vi "Hall of 6-Contact Sample Test.vi"(8 "error in (no error)":errorcluster) -> (0 "error out":errorcluster)   [LabVIEW 2016, in "Hall Effect Library.lvlib"]
uses:
  Hall Effect Library.lvlib
  Controls/Measurement.ctl
  Public/Controls/Data Items.ctl
  Public/Controls/Tests.ctl
  Global Variables/Test Settings.vi
  Global Variables/Hall Effect Data.vi
  Global Variables/Instrument Locations.vi
panel:
  out "Test Step":T1(ring)
  out "Measurement":T2
  out "Soak Until":timestamp
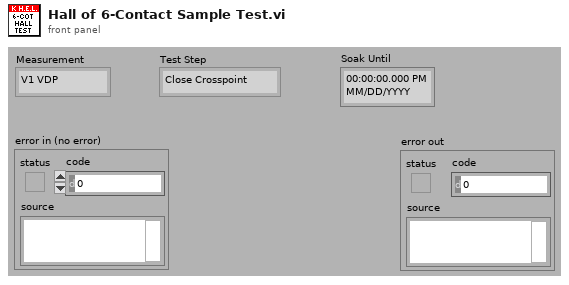
[diagram p1: front panel]
types:
  T1 = enum16{"Close Crosspoint", "Soak 1", "Zero Ammeter", "Zero Voltmeter", "I-SRC On", "Init Ammeter", "Soak 2", "Measure I", "Measure V", "I-SRC Off", "Open Crosspoint", "Done"}
  T2 = typedef "Hall Effect Library.lvlib/Measurement.ctl" = enum16{"V1 VDP", "V2 VDP", "V3 VDP", "V4 VDP", "V5 VDP", "V6 VDP", "V7 VDP", "V8 VDP", "V1 HE", "V2 HE", "V3 HE", "V4 HE", "V5 HE", "V6 HE", "V7 HE", "V8 HE", "V1 Res Bar", "V1 Hall Bar", "V1 Res 6-Cot", "V2 Res 6-Cot", "V3 Res 6-Cot", "V4 Res 6-Cot", "V1 Hall 6-Cot", "V2 Hall 6-Cot", "V3 Hall 6-Cot", "V4 Hall 6-Cot", "V5 Hall 6-Cot", "V6 Hall 6-Cot", "V7 Hall 6-Cot", "V8 Hall 6-Cot", "V1 Res 8-Cot", "V2 Res 8-Cot", "V3 Res 8-Cot", "V4 Res 8-Cot", "V1 Hall 8-Cot", "V2 Hall 8-Cot", "V3 Hall 8-Cot", "V4 Hall 8-Cot"}
  T3 = cluster{"RAvg":dbl, "RH1":dbl, "RH2":dbl, "uH":dbl}
  T4 = typedef "Hall Effect Library.lvlib/Resisitivity.ctl" = enum16{"Low", "High"}
  T5 = typedef "Hall Effect Library.lvlib/Tests.ctl" = enum16{"Van Der Pauw", "Hall Effect", "Bar Sample Resistivity", "Bar Sample Hall ", "6-Contact Sample Resistivity", "6-Contact Sample Hall", "8-Contact Sample Resistivity", "8-Contact Sample Hall", ""}
  T6 = typedef "Hall Effect Library.lvlib/Data Items.ctl" = enum16{"V1 Van Der Pauw", "V2 Van Der Pauw", "V3 Van Der Pauw", "V4 Van Der Pauw", "V5 Van Der Pauw", "V6 Van Der Pauw", "V7 Van Der Pauw", "V8 Van Der Pauw", "V1 Hall Effect", "V2 Hall Effect", "V3 Hall Effect", "V4 Hall Effect", "V5 Hall Effect", "V6  Hall Effect", "V7 Hall Effect", "V8 Hall Effect", "V1 Res Bar", "V1 Hall Bar", "V1 Res 6-Cot", "V2 Res 6-Cot", "V3 Res 6-Cot", "V4 Res 6-Cot", "V1 Hall 6-Cot", "V2 Hall 6-Cot", "V3 Hall 6-Cot", "V4 Hall 6-Cot", "V5 Hall 6-Cot", "V6 Hall 6-Cot", "V7 Hall 6-Cot", "V8 Hall 6-Cot", "V1 Res 8-Cot", "V2 Res 8-Cot", "V3 Res 8-Cot", "V4 Res 8-Cot", "V1 Hall 8-Cot", "V2 Hall 8-Cot", "V3 Hall 8-Cot", "V4 Hall 8-Cot", "Van Der Pauw Results", "Hall Effect Results", "Bar Sample Resistivity Results", "Bar Sample Hall Results", "6-Contact Resistivity Results", "6-Contact Hall Results", "8-Contact Resistivity Results", "8-Contact Hall Results"}
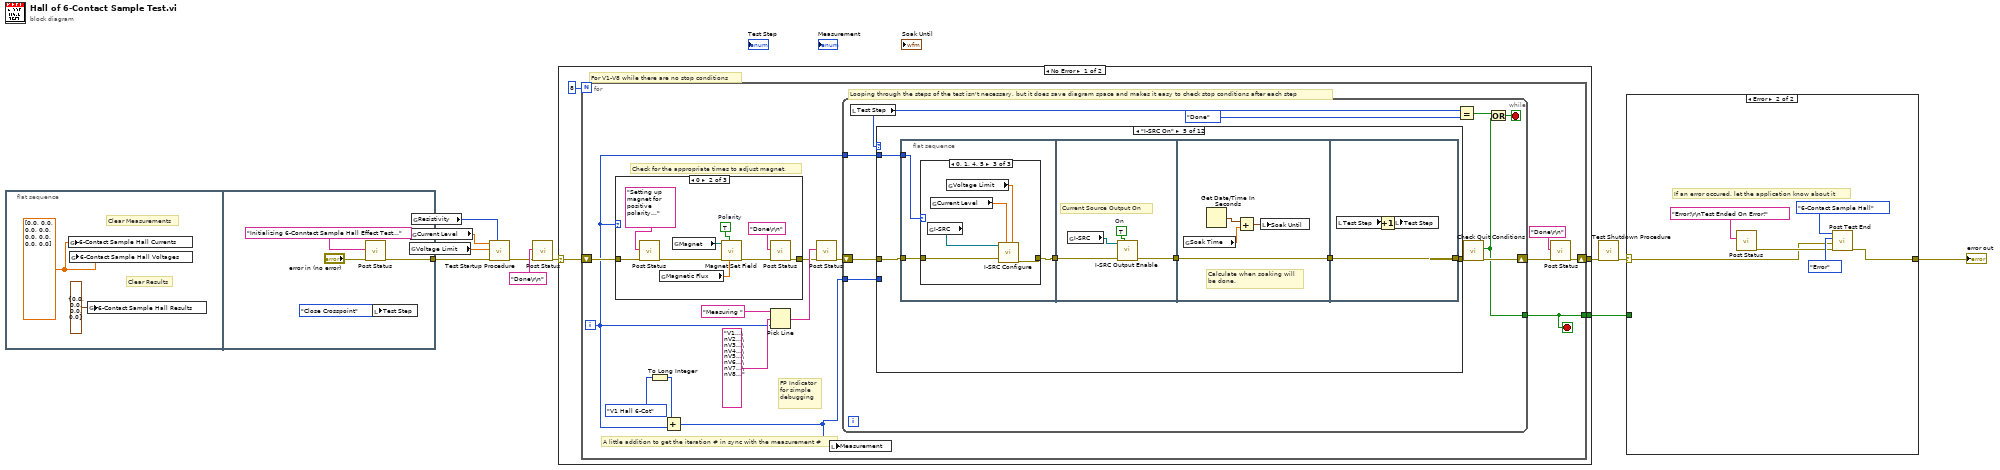
[diagram p0: block diagram]
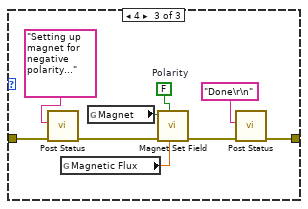
[diagram p3: hidden frame]
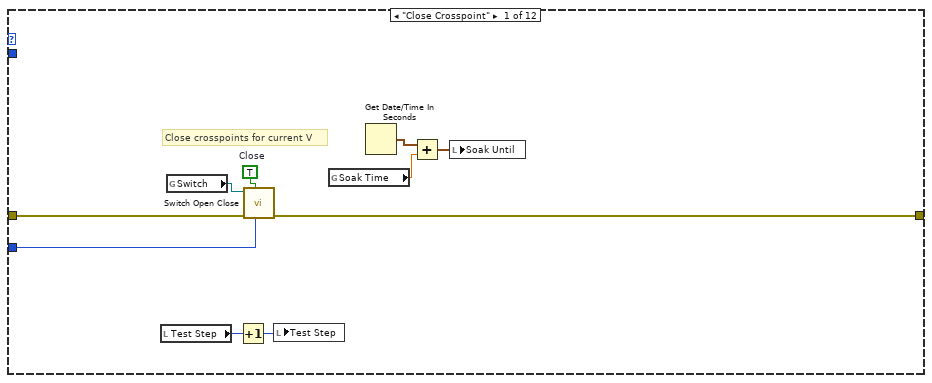
[diagram p4: hidden frame]
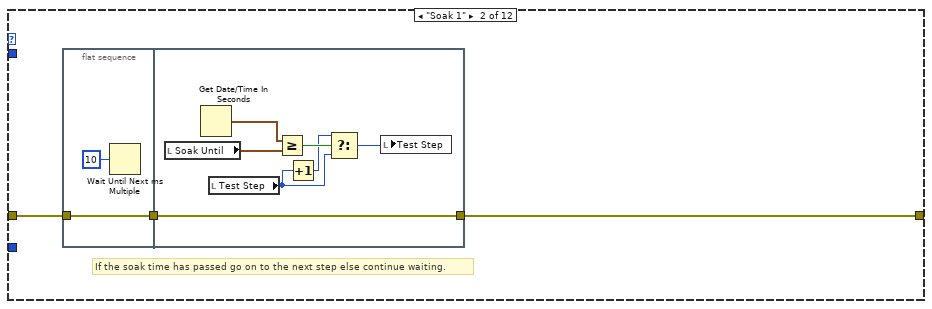
[diagram p5: hidden frame]
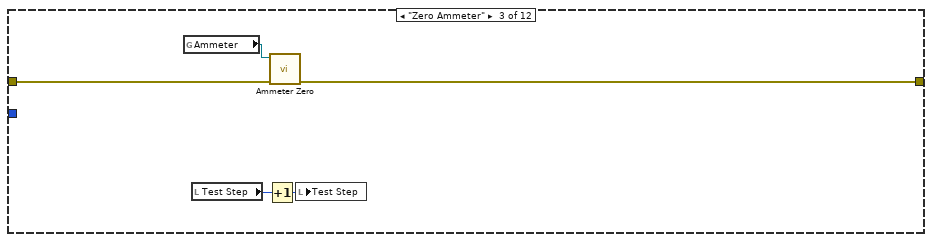
[diagram p6: hidden frame]
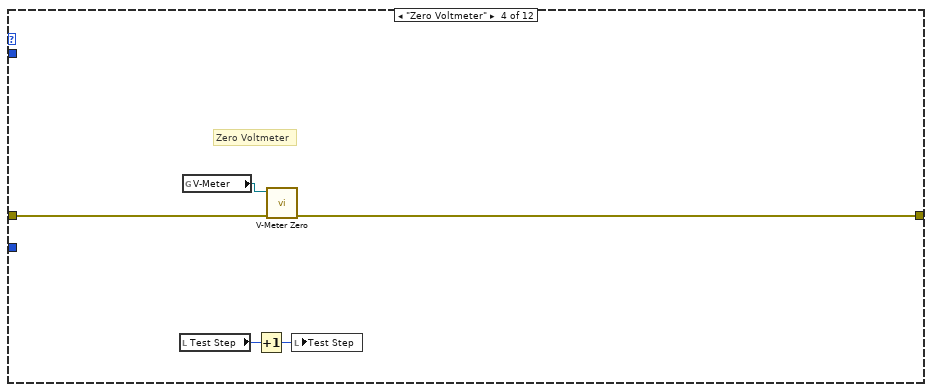
[diagram p7: hidden frame]
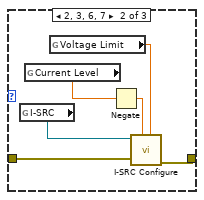
[diagram p9: hidden frame]
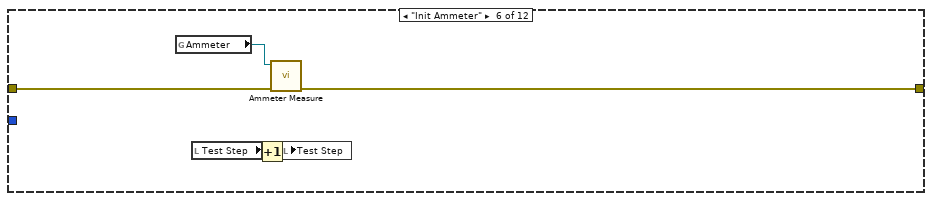
[diagram p10: hidden frame]
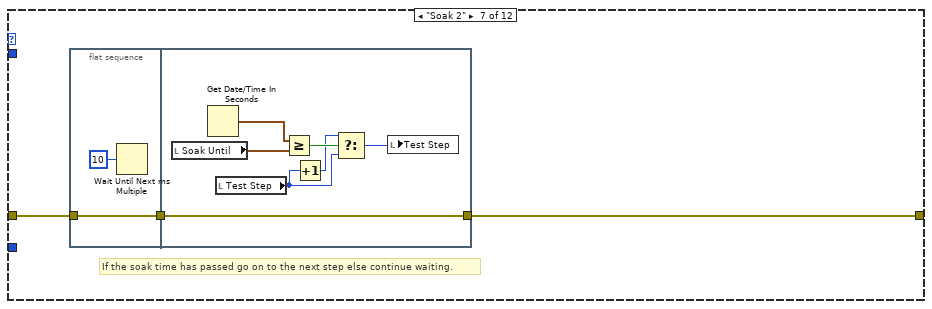
[diagram p11: hidden frame]
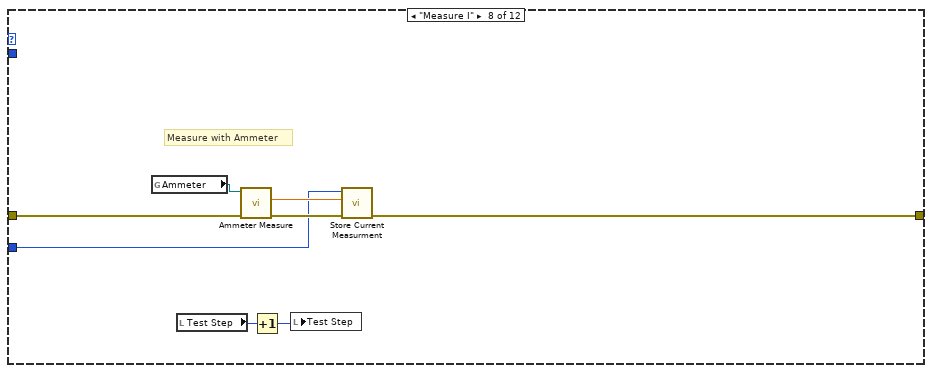
[diagram p12: hidden frame]
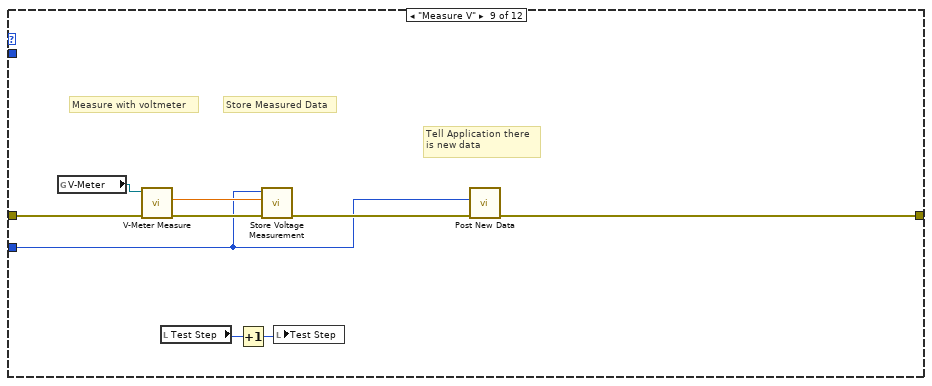
[diagram p13: hidden frame]
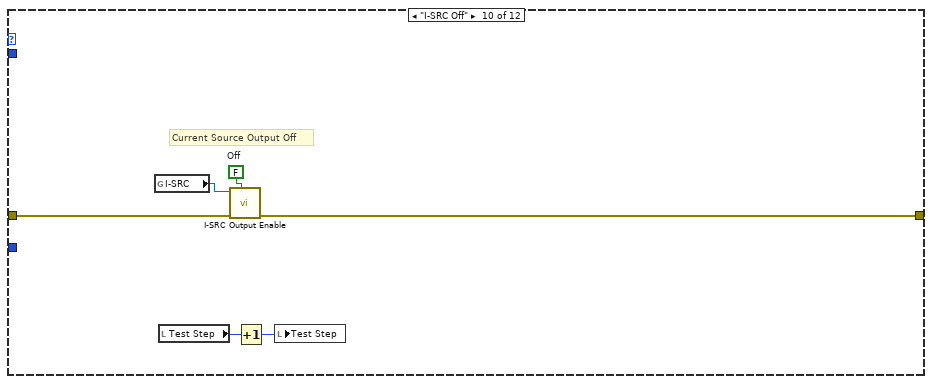
[diagram p14: hidden frame]
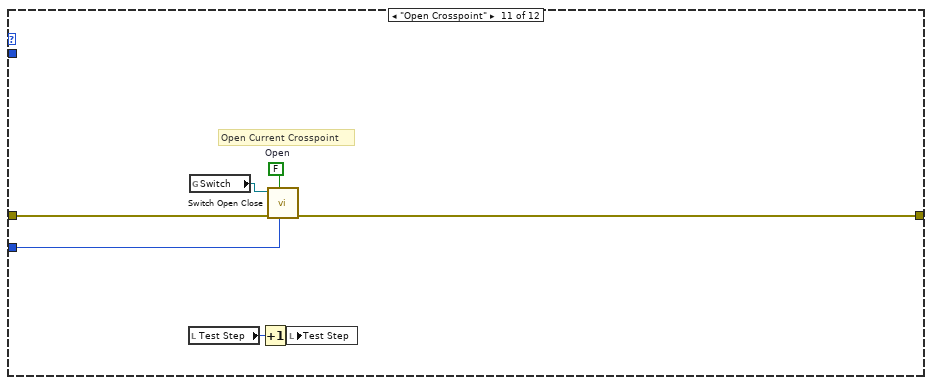
[diagram p15: hidden frame]
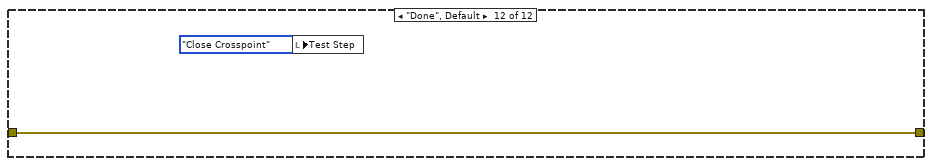
[diagram p16: hidden frame]
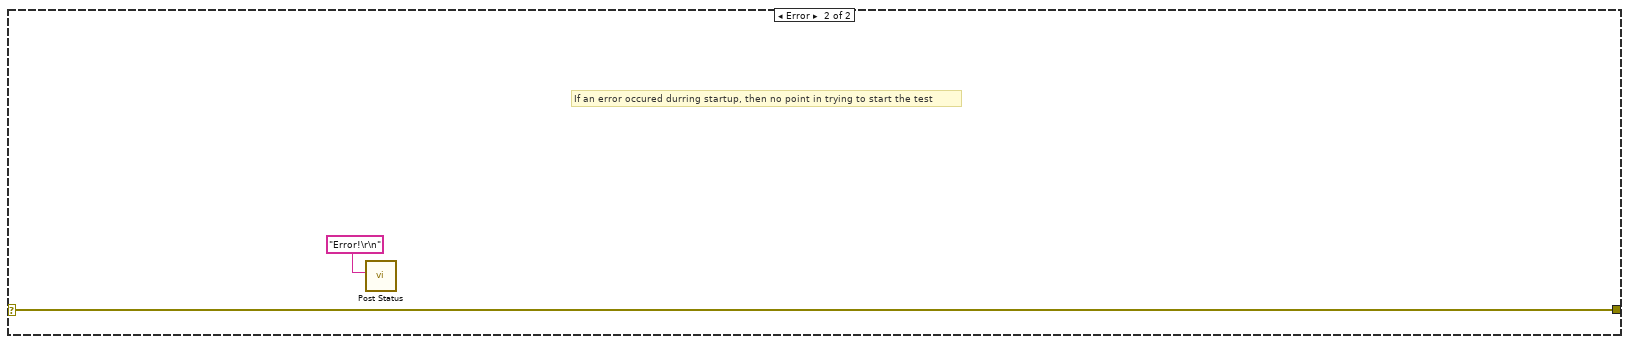
[diagram p17: hidden frame]
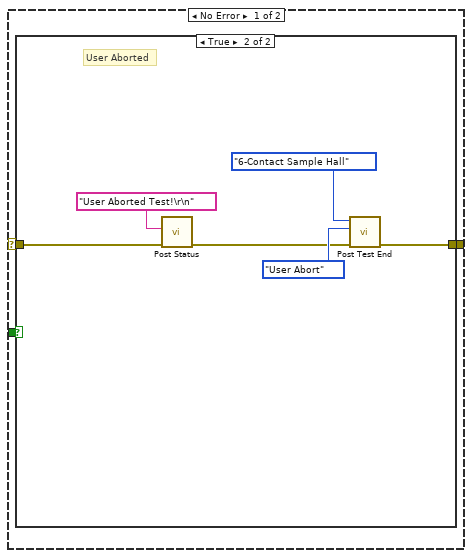
[diagram p18: hidden frame]
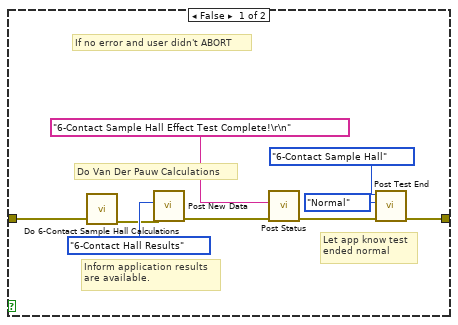
[diagram p19: hidden frame]
diagram:
  n1 = flat-sequence {
    tunnel: [w17] -> w5
    frame #0 {
      w12 = dbl[] [0.0, 0.0, 0.0, 0.0, 0.0, 0.0, 0.0, 0.0] ("6-Contact Sample Hall Voltages")
      # "Clear Results"
      # "Clear Measurements"
      n2 = global write "Hall Effect Data.vi" "6-Contact Sample Hall Currents"(w12) -> ()
      n3 = global write "Hall Effect Data.vi" "6-Contact Sample Hall Voltages"(w12) -> ()
      n4 = global write "Hall Effect Data.vi" "6-Contact Sample Hall Results"(T3 {"RAvg"=0.0, "RH1"=0.0, "RH2"=0.0, "uH"=0.0} ("6-Contact Sample Hall Results")) -> ()
    }
    frame #1 {
      n5 = call "Post Status.vi"("error in (no error)"="error in (no error)", "Status Message"="Initializing 6-Conntact Sample Hall Effect Test...") -> ("error out"=w17:errorcluster)  [unwired: 9 out]
      n6 = local write "Test Step"(T1."Close Crosspoint" ("Test Step")) -> ()
    }
  }
  n7 = global read "Test Settings.vi" "Voltage Limit"() -> (w6:dbl)
  n8 = global read "Test Settings.vi" "Current Level"() -> (w7:dbl)
  n9 = global read "Test Settings.vi" "Resistivity"() -> (w8:T4)
  n10 = call "Test Startup Procedure.vi"("Resistivity"=w8, "error in (no error)"=w5, "Voltage Limit"=w6, "Current Level"=w7) -> ("error out"=w3:errorcluster)  [unwired: 7 out]
  n11 = call "Post Status.vi"("error in (no error)"=w3, "Status Message"="Done\r\n") -> ("error out"=w9:errorcluster)  [unwired: 9 out]
  n12 = case shown="No Error" w9 {
    selector: w9 -> [w19 w179]
    tunnel: [w21 w179] -> w2
    tunnel: [w20 _] -> w10
    frame No Error {
      # "For V1-V8 while there are no stop conditions"
      n13 = for {
        N: 8 -> [_]
        shift-right: [w26] -> w21
        shift-left: w19 -> [w28]
        tunnel: [w23] -> w20
        i -> [w22]
        stop <- w23 stop-if-true
        # "A little addition to get the iteration # in sync with the measurement #"
        # "Check for the appropriate times to adjust magnet."
        # "FP Indicator\nfor simple\ndebugging"
        # "Looping through the steps of the test isn't necessary, but it does save diagram space and makes it easy to check stop conditions after each step"
        n14 = case shown="0" w22 {
          tunnel: [w36 w39 w47] -> w29
          tunnel: w28 -> [w36 w42 w51]
          frame Default {
          }
          frame 0 {
            w43 = TRUE  # Polarity
            n15 = call "Post Status.vi"("error in (no error)"=w42, "Status Message"="Setting up magnet for positive polarity...") -> ("error out"=w41:errorcluster)  [unwired: 9 out]
            n16 = global read "Test Settings.vi" "Magnetic Flux"() -> (w45:dbl)
            n17 = global read "Instrument Locations.vi" "Magnet"() -> (w44:refnum<visa-resource-name>)
            n18 = call "Magnet Set Field.vi"("Field Strength"=w45, "Polarity"=w43, "error in (no error)"=w41, "VISA resource name in"=w44) -> ("error out"=w40:errorcluster)  [unwired: 7 out]
            n19 = call "Post Status.vi"("error in (no error)"=w40, "Status Message"="Done\r\n") -> ("error out"=w39:errorcluster)  [unwired: 9 out]
          }
          frame 4 {
            w52 = FALSE  # Polarity
            n20 = call "Post Status.vi"("error in (no error)"=w51, "Status Message"="Setting up magnet for negative polarity...") -> ("error out"=w50:errorcluster)  [unwired: 9 out]
            n21 = global read "Test Settings.vi" "Magnetic Flux"() -> (w54:dbl)
            n22 = global read "Instrument Locations.vi" "Magnet"() -> (w53:refnum<visa-resource-name>)
            n23 = call "Magnet Set Field.vi"("Field Strength"=w54, "Polarity"=w52, "error in (no error)"=w50, "VISA resource name in"=w53) -> ("error out"=w48:errorcluster)  [unwired: 7 out]
            n24 = call "Post Status.vi"("error in (no error)"=w48, "Status Message"="Done\r\n") -> ("error out"=w47:errorcluster)  [unwired: 9 out]
          }
        }
        n25 = To Long Integer(number=Measurement."V1 Hall 6-Cot" ("Measurement")) -> (32bit integer=w31:i32)
        n26 = Add(x=w31, y=w22) -> (x+y=w24:i32)
        n27 = Pick Line(string ("")="Measuring ", multi-line string="V1...\nV2...\nV3...\nV4...\nV5...\nV6...\nV7...\nV8...", line index=w22) -> (output string=w33:string)
        n28 = call "Post Status.vi"("error in (no error)"=w29, "Status Message"=w33) -> ("error out"=w32:errorcluster)  [unwired: 9 out]
        n29 = local write "Measurement"(w24) -> ()
        n30 = while {
          shift-right: [w62] -> w25
          shift-left: w32 -> [w64]
          tunnel: w24 -> [w63]
          tunnel: [w58] -> w23
          tunnel: w22 -> [w55]
          stop <- w61 stop-if-true
          n31 = local read "Test Step"() -> (w59:T1)
          n32 = case shown="\"I-SRC On\"" w59 {
            tunnel: [w72 w75 w90 w94 w101 w132 w135 w150 w157 w165 w173 w177] -> w57
            tunnel: w64 -> [w71 w76 w91 w95 w102 w133 w136 w152 w161 w166 w172 w177]
            tunnel: w63 -> [w70 _ _ _ _ _ _ w148 w156 _ w171 _]
            tunnel: w55 -> [_ _ _ _ w97 _ _ _ _ _ _ _]
            frame "Close Crosspoint" {
              w73 = TRUE  # Close
              # "Close crosspoints for current V"
              n33 = local read "Test Step"() -> (w68:T1)
              n34 = global read "Instrument Locations.vi" "Switch"() -> (w74:refnum<visa-resource-name>)
              n35 = Increment(x=w68) -> (x+1=w69:T1)
              n36 = call "Switch Open Close.vi"("Measurement"=w70, "Open/Close (F: Open)"=w73, "error in (no error)"=w71, "VISA resource name in"=w74) -> ("error out"=w72:errorcluster)  [unwired: 7 out]
              n37 = local write "Test Step"(w69) -> ()
              n38 = global read "Test Settings.vi" "Soak Time"() -> (w66:dbl)
              n39 = Get Date/Time In Seconds() -> (seconds since 1Jan1904=w65:timestamp)
              n40 = Add(x=w65, y=w66) -> (x+y=w67:timestamp)
              n41 = local write "Soak Until"(w67) -> ()
            }
            frame "Soak 1" {
              # "If the soak time has passed go on to the next step else continue waiting."
              n42 = flat-sequence {
                tunnel: w76 -> [w78]
                tunnel: [w78] -> w77
                tunnel: [w82] -> w75
                tunnel: w77 -> [w82]
                frame #0 {
                  n43 = Wait Until Next ms Multiple(millisecond multiple=u32 10) -> ()  [unwired: 1 out]
                }
                frame #1 {
                  n44 = local read "Soak Until"() -> (w85:timestamp)
                  n45 = Get Date/Time In Seconds() -> (seconds since 1Jan1904=w86:timestamp)
                  n46 = local read "Test Step"() -> (w80:T1)
                  n47 = Greater Or Equal?(x=w86, y=w85) -> (x >= y?=w84:bool)
                  n48 = Increment(x=w80) -> (x+1=w81:T1)
                  n49 = Select(t=w81, s=w84, f=w80) -> (s? t:f=w83:T1)
                  n50 = local write "Test Step"(w83) -> ()
                }
              }
            }
            frame "Zero Ammeter" {
              n51 = global read "Instrument Locations.vi" "Ammeter"() -> (w89:refnum<visa-resource-name>)
              n52 = local read "Test Step"() -> (w87:T1)
              n53 = Increment(x=w87) -> (x+1=w88:T1)
              n54 = call "Ammeter Zero.vi"("error in (no error)"=w91, "VISA resource name in"=w89) -> ("error out"=w90:errorcluster)  [unwired: 9 out]
              n55 = local write "Test Step"(w88) -> ()
            }
            frame "Zero Voltmeter" {
              # "Zero Voltmeter"
              n56 = local read "Test Step"() -> (w93:T1)
              n57 = global read "Instrument Locations.vi" "V-Meter"() -> (w96:refnum<visa-resource-name>)
              n58 = Increment(x=w93) -> (x+1=w92:T1)
              n59 = call "V-Meter Zero.vi"("error in (no error)"=w95, "VISA resource name in"=w96) -> ("error out"=w94:errorcluster)  [unwired: 9 out]
              n60 = local write "Test Step"(w92) -> ()
            }
            frame "I-SRC On" {
              n61 = flat-sequence {
                tunnel: w102 -> [w104]
                tunnel: [w103] -> w98
                tunnel: w97 -> [w105]
                tunnel: [w118] -> w100
                tunnel: w98 -> [w119]
                tunnel: w100 -> [w125]
                tunnel: [w125] -> w99
                tunnel: [w128] -> w101
                tunnel: w99 -> [w128]
                frame #0 {
                  n62 = case shown="0, 1, 4, 5" w105 {
                    tunnel: w104 -> [w106 w111 w116]
                    tunnel: [w106 w110 w115] -> w103
                    frame Default {
                    }
                    frame 2, 3, 6, 7 {
                      n63 = global read "Instrument Locations.vi" "I-SRC"() -> (w112:refnum<visa-resource-name>)
                      n64 = global read "Test Settings.vi" "Current Level"() -> (w107:dbl)
                      n65 = global read "Test Settings.vi" "Voltage Limit"() -> (w109:dbl)
                      n66 = Negate(x=w107) -> (-x=w108:dbl)
                      n67 = call "I-SRC Configure.vi"("Voltage Limit"=w109, "Current Level"=w108, "error in (no error)"=w111, "VISA resource name in"=w112) -> ("error out"=w110:errorcluster)  [unwired: 6 in, 1 out]
                    }
                    frame 0, 1, 4, 5 {
                      n68 = global read "Instrument Locations.vi" "I-SRC"() -> (w117:refnum<visa-resource-name>)
                      n69 = global read "Test Settings.vi" "Current Level"() -> (w113:dbl)
                      n70 = global read "Test Settings.vi" "Voltage Limit"() -> (w114:dbl)
                      n71 = call "I-SRC Configure.vi"("Voltage Limit"=w114, "Current Level"=w113, "error in (no error)"=w116, "VISA resource name in"=w117) -> ("error out"=w115:errorcluster)  [unwired: 6 in, 1 out]
                    }
                  }
                }
                frame #1 {
                  w120 = TRUE  # On
                  # "Current Source Output On"
                  n72 = global read "Instrument Locations.vi" "I-SRC"() -> (w121:refnum<visa-resource-name>)
                  n73 = call "I-SRC Output Enable.vi"("Output (Off)"=w120, "error in (no error)"=w119, "VISA resource name in"=w121) -> ("error out"=w118:errorcluster)  [unwired: 8 out]
                }
                frame #2 {
                  # "Calculate when soaking will\nbe done."
                  n74 = global read "Test Settings.vi" "Soak Time"() -> (w123:dbl)
                  n75 = Get Date/Time In Seconds() -> (seconds since 1Jan1904=w122:timestamp)
                  n76 = Add(x=w122, y=w123) -> (x+y=w124:timestamp)
                  n77 = local write "Soak Until"(w124) -> ()
                }
                frame #3 {
                  n78 = local read "Test Step"() -> (w127:T1)
                  n79 = Increment(x=w127) -> (x+1=w126:T1)
                  n80 = local write "Test Step"(w126) -> ()
                }
              }
            }
            frame "Init Ammeter" {
              n81 = global read "Instrument Locations.vi" "Ammeter"() -> (w131:refnum<visa-resource-name>)
              n82 = local read "Test Step"() -> (w130:T1)
              n83 = Increment(x=w130) -> (x+1=w129:T1)
              n84 = call "Ammeter Measure.vi"("error in (no error)"=w133, "VISA resource name in"=w131) -> ("error out"=w132:errorcluster)  [unwired: 9 out]
              n85 = local write "Test Step"(w129) -> ()
            }
            frame "Soak 2" {
              # "If the soak time has passed go on to the next step else continue waiting."
              n86 = flat-sequence {
                tunnel: w136 -> [w137]
                tunnel: [w137] -> w134
                tunnel: [w141] -> w135
                tunnel: w134 -> [w141]
                frame #0 {
                  n87 = Wait Until Next ms Multiple(millisecond multiple=u32 10) -> ()  [unwired: 1 out]
                }
                frame #1 {
                  n88 = local read "Soak Until"() -> (w144:timestamp)
                  n89 = Get Date/Time In Seconds() -> (seconds since 1Jan1904=w145:timestamp)
                  n90 = local read "Test Step"() -> (w139:T1)
                  n91 = Greater Or Equal?(x=w145, y=w144) -> (x >= y?=w143:bool)
                  n92 = Increment(x=w139) -> (x+1=w140:T1)
                  n93 = Select(t=w140, s=w143, f=w139) -> (s? t:f=w142:T1)
                  n94 = local write "Test Step"(w142) -> ()
                }
              }
            }
            frame "Measure I" {
              # "Measure with Ammeter"
              n95 = global read "Instrument Locations.vi" "Ammeter"() -> (w153:refnum<visa-resource-name>)
              n96 = local read "Test Step"() -> (w147:T1)
              n97 = call "Ammeter Measure.vi"("error in (no error)"=w152, "VISA resource name in"=w153) -> ("error out"=w151:errorcluster, "Measurement"=w149:dbl)  [unwired: 8 out]
              n98 = Increment(x=w147) -> (x+1=w146:T1)
              n99 = local write "Test Step"(w146) -> ()
              n100 = call "Store Current Measurment.vi"("error in"=w151, "Value"=w149, "Measurement"=w148) -> ("error out"=w150:errorcluster)  [unwired: 8 out]
            }
            frame "Measure V" {
              # "Tell Application there\nis new data"
              # "Store Measured Data"
              # "Measure with voltmeter"
              n101 = global read "Instrument Locations.vi" "V-Meter"() -> (w162:refnum<visa-resource-name>)
              n102 = call "V-Meter Measure.vi"("error in (no error)"=w161, "VISA resource name in"=w162) -> ("error out"=w160:errorcluster, "Measurement"=w159:dbl)  [unwired: 1 in, 7 out]
              n103 = local read "Test Step"() -> (w154:T1)
              n104 = Increment(x=w154) -> (x+1=w155:T1)
              n105 = call "Store Voltage Measurement.vi"("error in"=w160, "Value"=w159, "Measurement"=w156) -> ("error out"=w158:errorcluster)  [unwired: 8 out]
              n106 = local write "Test Step"(w155) -> ()
              n107 = call "Post New Data.vi"("error in (no error)"=w158, "Data Item"=w156) -> ("error out"=w157:errorcluster)  [unwired: 9 out]
            }
            frame "I-SRC Off" {
              w167 = FALSE  # Off
              # "Current Source Output Off"
              n108 = global read "Instrument Locations.vi" "I-SRC"() -> (w168:refnum<visa-resource-name>)
              n109 = local read "Test Step"() -> (w164:T1)
              n110 = call "I-SRC Output Enable.vi"("Output (Off)"=w167, "error in (no error)"=w166, "VISA resource name in"=w168) -> ("error out"=w165:errorcluster)  [unwired: 8 out]
              n111 = Increment(x=w164) -> (x+1=w163:T1)
              n112 = local write "Test Step"(w163) -> ()
            }
            frame "Open Crosspoint" {
              w174 = FALSE  # Open
              # "Open Current Crosspoint"
              n113 = local read "Test Step"() -> (w170:T1)
              n114 = global read "Instrument Locations.vi" "Switch"() -> (w175:refnum<visa-resource-name>)
              n115 = Increment(x=w170) -> (x+1=w169:T1)
              n116 = call "Switch Open Close.vi"("Measurement"=w171, "Open/Close (F: Open)"=w174, "error in (no error)"=w172, "VISA resource name in"=w175) -> ("error out"=w173:errorcluster)  [unwired: 7 out]
              n117 = local write "Test Step"(w169) -> ()
            }
            frame "Done", Default {
              n118 = local write "Test Step"(T1."Close Crosspoint" ("Test Step")) -> ()
            }
          }
          n119 = Equal?(x=w59, y=T1."Done") -> (x = y?=w60:bool)
          n120 = call "Check Quit Conditions.vi"("error in (no error)"=w57) -> ("error out"=w62:errorcluster, "Quit?"=w58:bool)  [unwired: 9 out]
          n121 = Or(x=w60, y=w58) -> (x .or. y?=w61:bool)
        }
        n122 = call "Post Status.vi"("error in (no error)"=w25, "Status Message"="Done\r\n") -> ("error out"=w26:errorcluster)  [unwired: 9 out]
      }
    }
    frame Error {
      # "If an error occured durring startup, then no point in trying to start the test"
      n123 = call "Post Status.vi"("Status Message"="Error!\r\n") -> ()  [unwired: 1 in, 10 out]
    }
  }
  n124 = call "Test Shutdown Procedure.vi"("error in (no error)"=w2) -> ("error out"=w1:errorcluster)  [unwired: 10 out]
  n125 = case shown="Error" w1 {
    selector: w1 -> [w181 w199]
    tunnel: w10 -> [w182 _]
    tunnel: [w180 w200] -> w11
    frame No Error {
      n126 = case shown="True" w182 {
        tunnel: w181 -> [w184 w196]
        tunnel: [w186 w193] -> w180
        frame False {
          # "Let app know test\nended normal"
          # "Inform application results\nare available."
          # "Do Van Der Pauw Calculations"
          # "If no error and user didn't ABORT"
          n127 = call "Do 6-Contact Sample Hall Calculations.vi"("error in (no error)"=w184) -> ("error out"=w183:errorcluster)  [unwired: 10 in]
          n128 = call "Post New Data.vi"("error in (no error)"=w183, "Data Item"=Data_Items."6-Contact Hall Results") -> ("error out"=w189:errorcluster)  [unwired: 9 out]
          n129 = call "Post Status.vi"("error in (no error)"=w189, "Status Message"="6-Contact Sample Hall Effect Test Complete!\r\n") -> ("error out"=w188:errorcluster)  [unwired: 9 out]
          n130 = call "Post Test End.vi"("error in (no error)"=w188, "Test End"=enum16{"Normal", "User Abort", "Error"}."Normal", "Test"=Tests."6-Contact Sample Hall") -> ("error out"=w186:errorcluster)  [unwired: 1 in, 7 out]
        }
        frame True {
          # "User Aborted"
          n131 = call "Post Status.vi"("error in (no error)"=w196, "Status Message"="User Aborted Test!\r\n") -> ("error out"=w195:errorcluster)  [unwired: 9 out]
          n132 = call "Post Test End.vi"("error in (no error)"=w195, "Test End"=enum16{"Normal", "User Abort", "Error"}."User Abort", "Test"=Tests."6-Contact Sample Hall") -> ("error out"=w193:errorcluster)  [unwired: 1 in, 7 out]
        }
      }
    }
    frame Error {
      # "If an error occured, let the application know about it"
      n133 = call "Post Status.vi"("Status Message"="Error!\r\nTest Ended On Error!") -> ("error out"=w202:errorcluster)  [unwired: 1 in, 9 out]
      n134 = call "Post Test End.vi"("error in (no error)"=w202, "Test End Error (no error)"=w199, "Test End"=enum16{"Normal", "User Abort", "Error"}."Error", "Test"=Tests."6-Contact Sample Hall") -> ("error out"=w200:errorcluster)  [unwired: 7 out]
    }
  }
  "error out" <- w11
